vi "Interface_Asset_Get Parameter Control Refs.vi"(8 "error in (no error)":errorcluster, 11 "Grid in":refnum<class "Grid.lvclass">) -> (0 "error out":errorcluster, 2 "Controls[]":refnum<vi>[](array[refnum]), 3 "Grid out":refnum<class "Grid.lvclass">)   [LabVIEW 2015, in "Grid.lvclass"]
uses:
  Grid.lvclass
  Grid_Status.ctl
  Grid.lvclass/Grid.ctl
panel:
  out "Status":T1
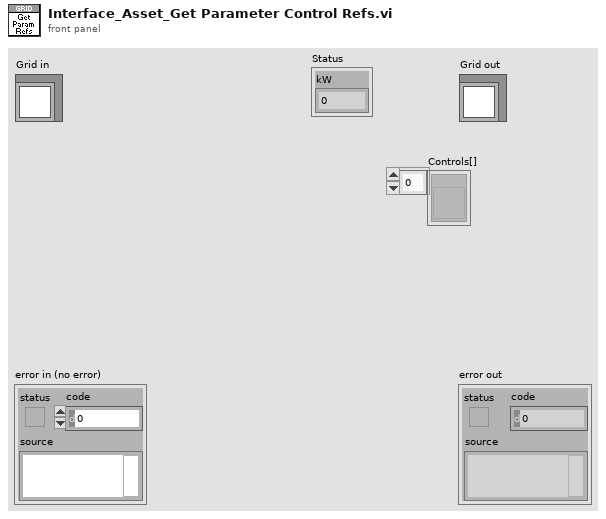
[diagram p1: front panel]
types:
  T1 = typedef "Grid.lvclass/Grid_Status.ctl" = cluster{"kW":dbl}
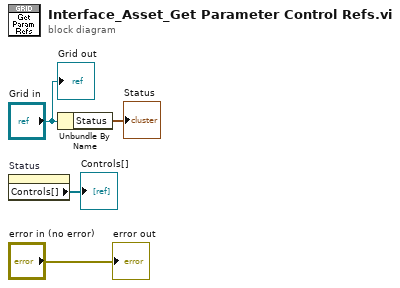
[diagram p0: block diagram]
diagram:
  n1 = property on="Status" class="Clust (strict)"() -> ("Controls[]"=→"Controls[]":refnum<vi>[])  [unwired: 2 in, 2 out]
  n2 = Unbundle By Name("Grid in") -> ("Status"=→"Status":T1)
  "error out" <- "error in (no error)"
  "Grid out" <- "Grid in"
